vi "Configure Trigger Signal.vi"(0 "VISA resource name":refnum<visa-resource-name>, 1 "Trigger Mode (1: Key)":i32(ring)=1 items=["Immediate", "Key", "Ext", "Bus", "Aux I/O"], 2 "Aux IO Trigger Polarity (0: Positive)":i32(ring) items=["Positive", "Negative"], 5 "Enable Trigger Delay (F: Disable)":bool, 7 "Delay Bits (0)":u32, 9 "Cycle Count (1)":u32=1, 11 "error in (no error)":errorcluster, 12 "External Trigger Source (0: Trigger1)":i32(ring) items=["Trigger1", "Trigger2", "Pulse"]) -> (4 "VISA resource name out":refnum<visa-resource-name>, 15 "error out":errorcluster)   [LabVIEW 2018, in "Agilent PSG MXG Series.lvlib"]
doc: "Configures trigger signal for the bit error rate test (BERT) measurements.\n\n<b>Note:</b>\nIt is applicable for N5172B/82B with <b>Option UN7</b> only."
uses:
  Agilent PSG MXG Series.lvlib
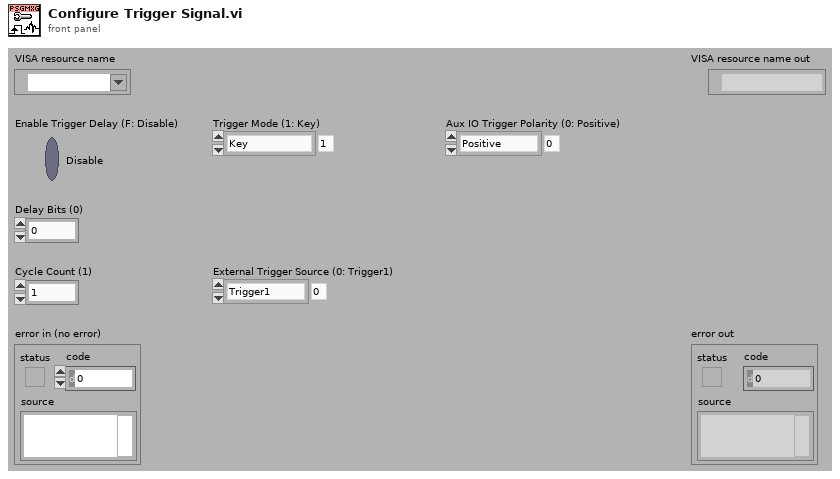
[diagram p1: front panel]
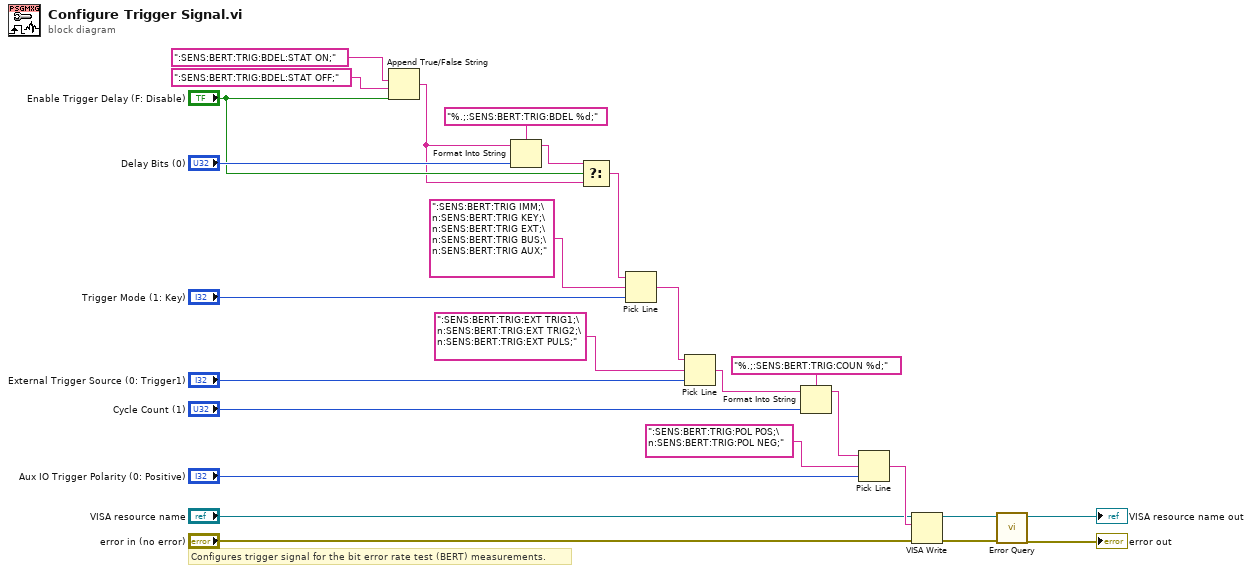
[diagram p0: block diagram]
diagram:
  # "Configures trigger signal for the bit error rate test (BERT) measurements."
  n1 = Append True/False String(1:"Enable Trigger Delay (F: Disable)", 2:":SENS:BERT:TRIG:BDEL:STAT OFF;", 3:":SENS:BERT:TRIG:BDEL:STAT ON;") -> (0:w3:string)  [unwired: 1 in]
  n2 = Format Into String(format string="%.;:SENS:BERT:TRIG:BDEL %d;", initial string=w3, "Delay Bits (0)") -> (resulting string=w4:string)  [unwired: 1 in, 1 out]
  n3 = Select(t=w4, s="Enable Trigger Delay (F: Disable)", f=w3) -> (s? t:f=w2:string)
  n4 = Pick Line(string ("")=w2, multi-line string=":SENS:BERT:TRIG IMM;\n:SENS:BERT:TRIG KEY;\n:SENS:BERT:TRIG EXT;\n:SENS:BERT:TRIG BUS;\n:SENS:BERT:TRIG AUX;", line index="Trigger Mode (1: Key)") -> (output string=w20:string)
  n5 = Pick Line(string ("")=w20, multi-line string=":SENS:BERT:TRIG:EXT TRIG1;\n:SENS:BERT:TRIG:EXT TRIG2;\n:SENS:BERT:TRIG:EXT PULS;", line index="External Trigger Source (0: Trigger1)") -> (output string=w1:string)
  n6 = Format Into String(format string="%.;:SENS:BERT:TRIG:COUN %d;", initial string=w1, "Cycle Count (1)") -> (resulting string=w13:string)  [unwired: 1 in, 1 out]
  n7 = Pick Line(string ("")=w13, multi-line string=":SENS:BERT:TRIG:POL POS;\n:SENS:BERT:TRIG:POL NEG;", line index="Aux IO Trigger Polarity (0: Positive)") -> (output string=w12:string)
  n8 = VISA Write(VISA resource name="VISA resource name", write buffer=w12, error in (no error)="error in (no error)") -> (VISA resource name out=w9:refnum<visa-resource-name>, error out=w8:errorcluster)  [unwired: 1 out]
  n9 = call "Error Query.vi"("error in (no error)"=w8, "VISA resource name"=w9) -> ("error out"=→"error out":errorcluster, "VISA resource name out"=→"VISA resource name out":refnum<visa-resource-name>)  [unwired: 6 in, 2 out]
